vi "Get Job Data.vi"(0 "SystemLink repo in":T3, 5 "job ID":string, 11 "error in (no error)":errorcluster) -> (4 "SystemLink repo out":T3, 6 "job data":T1, 15 "error out":errorcluster)   [LabVIEW 2017, in "SystemLink_Repo_API.lvlib"]
doc: "Returns the job data for the specified job ID."
uses:
  SystemLink_Repo_API.lvlib
  systemlink repo.ctl
  <vilib>/httpClient/ClientHandle.ctl
  syslink_job.ctl
  syslink_job_datatype.ctl
  5f630843-bab1-4963-9217-30a19a5e7c60.vi
  8083b1b1-7765-49a7-b76a-f1cdae8dcbd0.vi
  <vilib>/Utility/error.llb/Trim Whitespace One-Sided.vi
  <vilib>/JDP Science/JSONtext/JSON text to Variant.vi
  <vilib>/JDP Science/JSONtext/LVClass Serializer/JSONtext LVClass Serializer.lvclass
  <vilib>/httpClient/LabVIEWHTTPClient.lvlib
panel:
  out "resulting string":string
  out "body":string
  out "headers":string
  # "Status will be \"SUCCEEDED\" for a successful job and \"FAILED\" for a failed job."
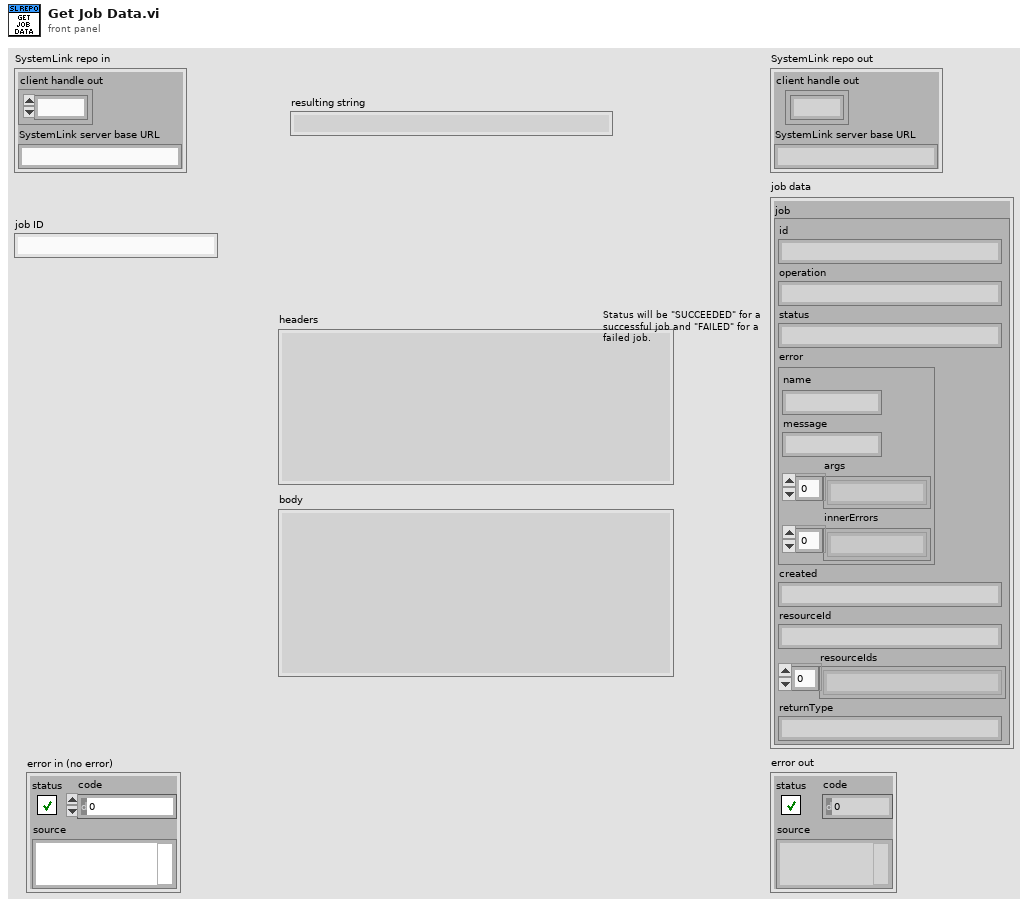
[diagram p1: front panel]
types:
  T1 = typedef "SystemLink_Repo_API.lvlib/syslink_job.ctl" = cluster{"job":T2}
  T2 = typedef "SystemLink_Repo_API.lvlib/syslink_job_datatype.ctl" = cluster{"id":string, "operation":string, "status":string, "error":cluster{"name":string, "message":string, "args":string[], "innerErrors":string[]}, "created":string, "resourceId":string, "resourceIds":string[], "returnType":string}
  T3 = typedef "SystemLink_Repo_API.lvlib/systemlink repo.ctl" = cluster{"client handle out":T4, "SystemLink server base URL":string}
  T4 = typedef "LabVIEWHTTPClient.lvlib/ClientHandle.ctl" = refnum<k1>
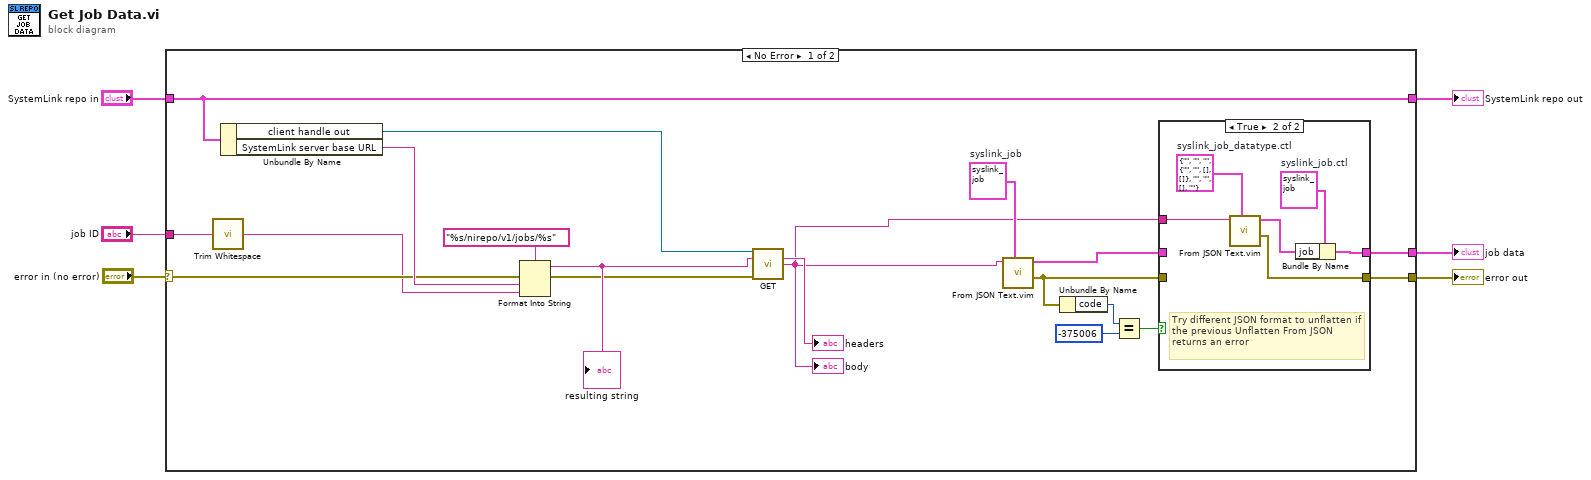
[diagram p0: block diagram]
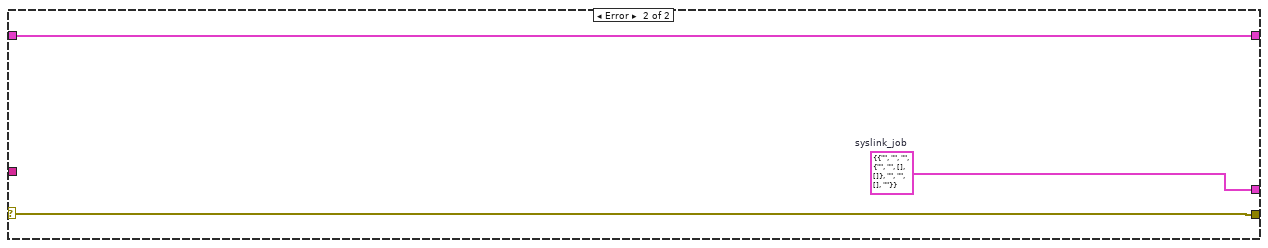
[diagram p3: hidden frame]
diagram:
  n1 = case shown="No Error" "error in (no error)" {
    selector: "error in (no error)" -> [w21 w36]
    tunnel: "SystemLink repo in" -> [w17 w34]
    tunnel: [w10 w36] -> w5
    tunnel: "job ID" -> [w18 _]
    tunnel: [w12 w35] -> w1
    tunnel: [w17 w34] -> w2
    frame No Error {
      w8 = T1 {"job"={"id"="", "operation"="", "status"="", "error"={"name"="", "message"="", "args"=[], "innerErrors"=[]}, "created"="", "resourceId"="", "resourceIds"=[], "returnType"=""}}  # syslink_job
      n2 = call <vilib>:"Trim Whitespace.vi"("string"=w18) -> ("trimmed string"=w19:string)  [unwired: 1 in]
      n3 = Unbundle By Name(w17) -> ("client handle out"=w9:T4, "SystemLink server base URL"=w22:string)
      n4 = Format Into String(format string="%s/nirepo/v1/jobs/%s", error in=w21, w22, w19) -> (resulting string=w23:string, error out=w20:errorcluster)  [unwired: 1 in]
      "resulting string" <- w23
      n5 = call <vilib>:"GET.vi"("client handle"=w9, "url"=w23, "error in (no error)"=w20) -> ("headers"=→"headers":string, "body"=w7:string)  [unwired: 9 in, 2 out]
      "body" <- w7
      n6 = call "From JSON Text.vim"("Data Type and Default Value"=w8, "JSON"=w7) -> ("error out"=w11:errorcluster, "Data out"=w13:T1)  [unwired: 8 in]
      n7 = Unbundle By Name(w11) -> ("code"=w16:i32)
      n8 = Equal?(x=w16, y=-375006) -> (x = y?=w14:bool)
      n9 = case shown="True" w14 {
        tunnel: w13 -> [w27 _]
        tunnel: [w27 w30] -> w12
        tunnel: w11 -> [w26 _]
        tunnel: [w26 w29] -> w10
        tunnel: w7 -> [_ w33]
        frame False {
        }
        frame True {
          w32 = T1 {"job"={"id"="", "operation"="", "status"="", "error"={"name"="", "message"="", "args"=[], "innerErrors"=[]}, "created"="", "resourceId"="", "resourceIds"=[], "returnType"=""}}  # syslink_job.ctl
          w28 = T2 {"id"="", "operation"="", "status"="", "error"={"name"="", "message"="", "args"=[], "innerErrors"=[]}, "created"="", "resourceId"="", "resourceIds"=[], "returnType"=""}  # syslink_job_datatype.ctl
          # "Try different JSON format to unflatten if the previous Unflatten From JSON returns an error"
          n10 = call "From JSON Text.vim"("Data Type and Default Value"=w28, "JSON"=w33) -> ("error out"=w29:errorcluster, "Data out"=w31:T2)  [unwired: 8 in]
          n11 = Bundle By Name(cluster=w32, "job"=w31) -> (w30:T1)
        }
      }
    }
    frame Error {
      w35 = T1 {"job"={"id"="", "operation"="", "status"="", "error"={"name"="", "message"="", "args"=[], "innerErrors"=[]}, "created"="", "resourceId"="", "resourceIds"=[], "returnType"=""}}  # syslink_job
    }
  }
  "error out" <- w5
  "SystemLink repo out" <- w2
  "job data" <- w1
